vi "IB_2019_2018_RW_Convert_Path_to_Relative.vi"(8 "error in (no error)":errorcluster, 10 "commonPath":path, 11 "absolutePath":path) -> (0 "error out":errorcluster, 2 "relativeType":T1, 3 "newPath":path)   [LabVIEW 2020]
uses:
  <vilib>/AppBuilder/IB_RW_Project/IB_Relative_Path_Type.ctl
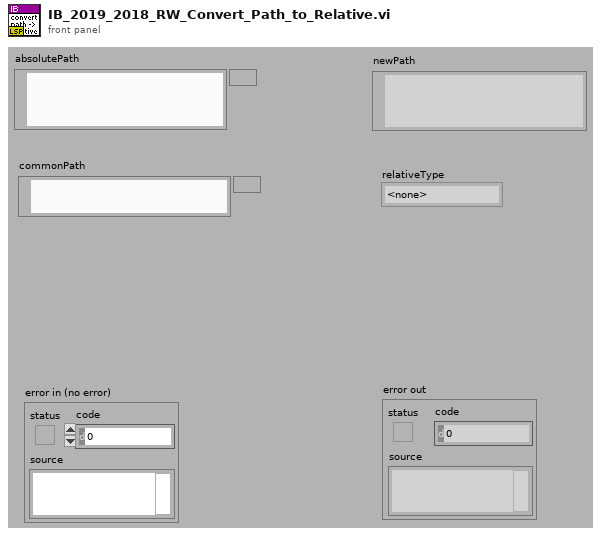
[diagram p1: front panel]
types:
  T1 = typedef "IB_Relative_Path_Type.ctl" = enum16{"<none>", "relativeToCommon", "relativeToAppDir", "relativeToProject"}
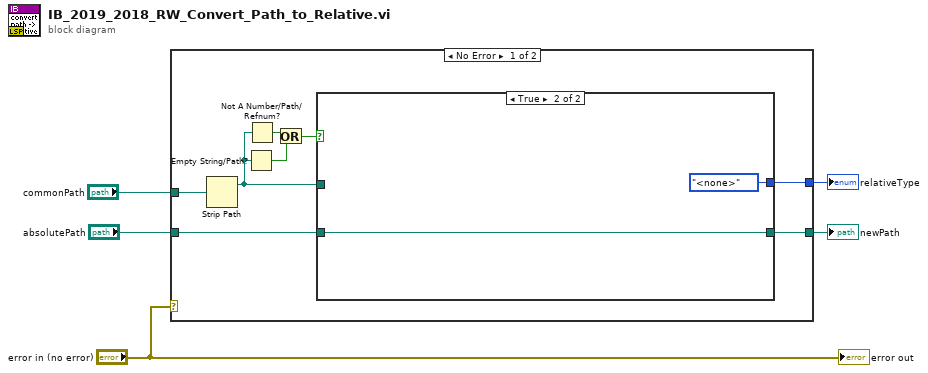
[diagram p0: block diagram]
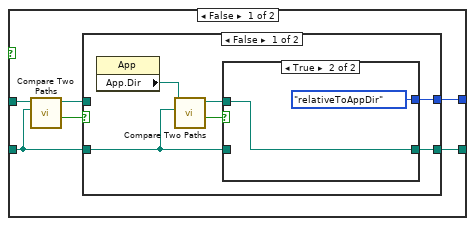
[diagram p2: hidden frame]
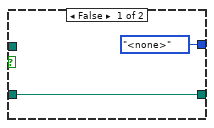
[diagram p3: hidden frame]
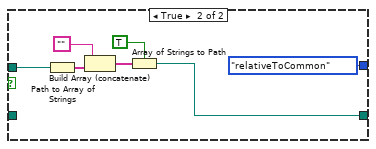
[diagram p4: hidden frame]
diagram:
  n1 = case shown="No Error" "error in (no error)" {
    tunnel: "commonPath" -> [w6 _]
    tunnel: "absolutePath" -> [w13 w39]
    tunnel: [w12 w39] -> w3
    tunnel: [w11 _] -> w2
    frame No Error {
      n2 = Strip Path(path=w6) -> (stripped path=w10:path)  [unwired: 1 out]
      n3 = Empty String/Path?(string/path=w10) -> (empty?=w8:bool)
      n4 = Not A Number/Path/Refnum?(number/path/refnum=w10) -> (NaN/Path/Refnum?=w9:bool)
      n5 = Or(x=w9, y=w8) -> (x .or. y?=w7:bool)
      n6 = case shown="True" w7 {
        tunnel: w13 -> [w18 w38]
        tunnel: [w17 w38] -> w12
        tunnel: [w16 IB_Relative_Path_Type."<none>" ("relativeType")] -> w11
        tunnel: w10 -> [w14 _]
        frame False {
          n7 = call <vilib>:"Compare Two Paths.vi"("Path 2"=w18, "Path 1"=w14) -> ("Path 2 Relative to Path 1?"=w19:bool, "Relative Path from 1 to 2"=w15:path)  [unwired: 6 in, 2 out]
          n8 = case shown="False" w19 {
            tunnel: w18 -> [w22 _]
            tunnel: [w23 w30] -> w17
            tunnel: [w20 IB_Relative_Path_Type."relativeToCommon" ("relativeType")] -> w16
            tunnel: w15 -> [_ w35]
            frame False {
              n9 = property class="App"() -> ("App.Dir"=w25:path)  [unwired: 2 in, 2 out]
              n10 = call <vilib>:"Compare Two Paths.vi"("Path 2"=w22, "Path 1"=w25) -> ("Path 2 Relative to Path 1?"=w24:bool, "Relative Path from 1 to 2"=w21:path)  [unwired: 6 in, 2 out]
              n11 = case shown="True" w24 {
                tunnel: [w27 w29] -> w23
                tunnel: w22 -> [w27 _]
                tunnel: w21 -> [_ w29]
                tunnel: [IB_Relative_Path_Type."<none>" ("relativeType") IB_Relative_Path_Type."relativeToAppDir" ("relativeType")] -> w20
                frame False {
                }
                frame True {
                }
              }
            }
            frame True {
              n12 = Path to Array of Strings(0:w35) -> (2:w34:string[])  [unwired: 1 out]
              n13 = Build Array (concatenate)("", w34) -> (w32:string[])
              n14 = Array of Strings to Path(0:w32, 1:TRUE ("relative")) -> (2:w30:path)
            }
          }
        }
        frame True {
        }
      }
    }
    frame Error {
    }
  }
  "newPath" <- w3
  "relativeType" <- w2
  "error out" <- "error in (no error)"
